vi "Producto inventario.vi"(8 "error in (no error)":errorcluster, 10 "Productos inventario":i32, 11 "Soda Actor in":refnum<class "Soda Actor.lvclass">) -> (0 "error out":errorcluster, 3 "Soda Actor out":refnum<class "Soda Actor.lvclass">)   [LabVIEW 2020, in "Soda Actor.lvlib" / "Soda Actor.lvclass"]
uses:
  Soda Actor.lvclass
  Soda Actor.lvclass/Soda Actor.ctl
  <vilib>/Utility/config.llb/Read Key (Double).vi
  <vilib>/Utility/config.llb/Write Key (String).vi
  <vilib>/Utility/config.llb/Read Key (String).vi
  <vilib>/Utility/config.llb/NI_LVConfig.lvlib
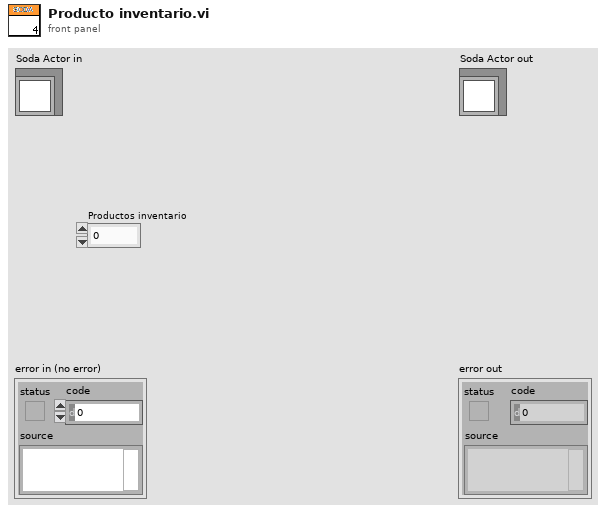
[diagram p1: front panel]
types:
  T1 = typedef "NI_LVConfig.lvlib/Config Data RefNum.ctl" = refnum<k1>
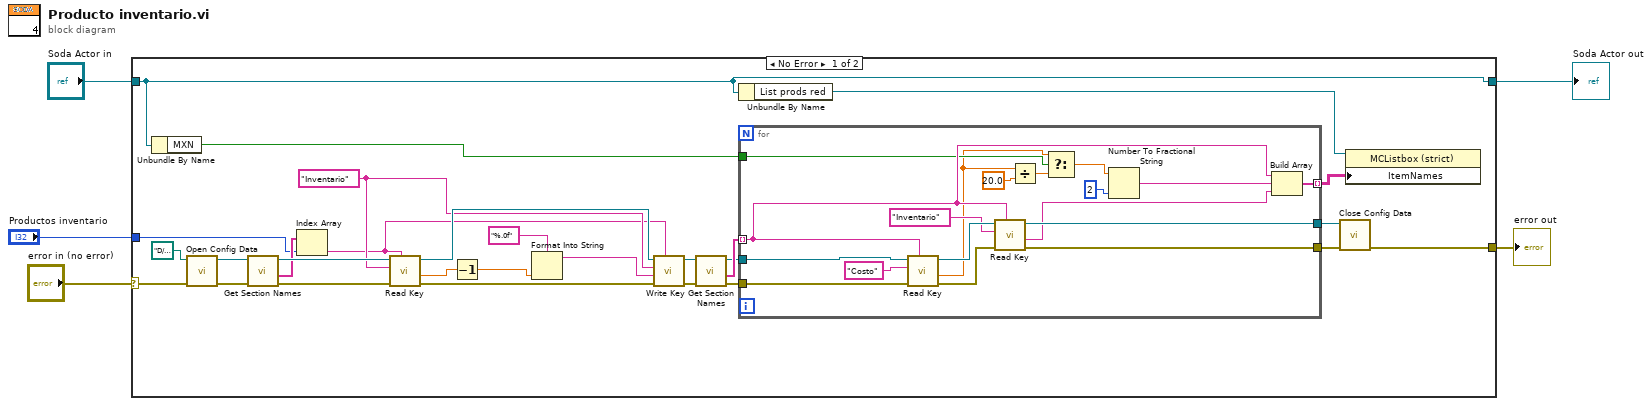
[diagram p0: block diagram]
diagram:
  n1 = case shown="No Error" "error in (no error)" {
    selector: "error in (no error)" -> [w29 w53]
    tunnel: [w7 w53] -> w4
    tunnel: [w9 w52] -> w2
    tunnel: "Soda Actor in" -> [w9 w52]
    tunnel: "Productos inventario" -> [w27 _]
    frame No Error {
      w20 = "Inventario" ("key")
      n2 = Unbundle By Name(w9) -> ("MXN"=w8:bool)
      n3 = call <vilib>:"Open Config Data.vi"("error in (no error)"=w29, "configuration file path"=path "D:/fork/Maquina-Expendedora/maquina/Soda Actor.ini") -> ("error out"=w33:errorcluster, "refnum"=w32:T1)  [unwired: 7 in, 1 out]
      n4 = call <vilib>:"Get Section Names.vi"("error in (no error)"=w33, "refnum"=w32) -> ("error out"=w25:errorcluster, "section names"=w28:string[], "refnum out"=w31:T1)  [unwired: 7 in]
      n5 = Index Array "Index Array"(array=w28, index=w27) -> (element=w6:string)
      n6 = call-poly <vilib>:"Read Key.vi"("section"=w6, "error in (no error)"=w25, "key"=w20, "refnum"=w31) -> ("error out"=w19:errorcluster, "value"=w26:dbl, "refnum out"=w21:T1)  [unwired: 4 in, 1 out]
      n7 = Decrement(x=w26) -> (x-1=w23:dbl)
      n8 = Format Into String "Format Into String"(format string="%.0f", w23) -> (resulting string=w22:string)  [unwired: 2 in, 1 out]
      n9 = call-poly <vilib>:"Write Key.vi"("section"=w6, "error in (no error)"=w19, "value"=w22, "key"=w20, "refnum"=w21) -> ("error out"=w18:errorcluster, "refnum out"=w17:T1)  [unwired: 4 in, 1 out]
      n10 = call <vilib>:"Get Section Names.vi"("error in (no error)"=w18, "refnum"=w17) -> ("error out"=w16:errorcluster, "section names"=w15:string[], "refnum out"=w14:T1)  [unwired: 7 in]
      n11 = Unbundle By Name(w9) -> ("List prods red"=w10:refnum<vi>)
      n12 = for {
        tunnel: w14 -> [w51]
        tunnel: w16 -> [w50]
        tunnel: [w47] -> w13
        tunnel: [w46] -> w12
        tunnel: w8 -> [w38]
        tunnel: w15 -> [w43] mode=indexing
        tunnel: [w41] -> w11 mode=indexing
        n13 = call-poly <vilib>:"Read Key.vi"("section"=w43, "error in (no error)"=w50, "key"="Costo", "refnum"=w51) -> ("error out"=w49:errorcluster, "value"=w36:dbl, "refnum out"=w48:T1)  [unwired: 4 in, 1 out]
        n14 = call-poly <vilib>:"Read Key.vi"("section"=w43, "error in (no error)"=w49, "key"="Inventario", "refnum"=w48) -> ("error out"=w47:errorcluster, "value"=w42:string, "refnum out"=w46:T1)  [unwired: 4 in, 1 out]
        n15 = Divide(x=w36, y=20.0) -> (x/y=w34:dbl)
        n16 = Select(t=w36, s=w38, f=w34) -> (s? t:f=w37:dbl)
        n17 = Number To Fractional String(number=w37, precision (6)=i16 2) -> (F-format string=w40:string)  [unwired: 2 in]
        n18 = Build Array(w43, w40, w42) -> (w41:string[])
      }
      n19 = call <vilib>:"Close Config Data.vi"("error in (no error)"=w13, "refnum"=w12) -> ("error out"=w7:errorcluster)  [unwired: 8 in, 1 out]
      n20 = property class="MCListbox (strict)"(reference=w10, "ItemNames"=w11) -> ()  [unwired: 1 in, 2 out]
    }
    frame Error {
    }
  }
  "error out" <- w4
  "Soda Actor out" <- w2
